vi "solar_voy TCP Listener Wait.vi"(7 "Instance":i32, 8 "error in (no error)":errorcluster, 9 "timeout ms (-1)":i32=-1, 10 "Listener ID":refnum<k5>, 11 "Voyager Refnum in":T1) -> (0 "error out":errorcluster, 2 "Connection ID":refnum<k5>, 3 "Voyager Refnum out":T1)   [LabVIEW 2018]
doc: "This waits for a single TCP client connection."
uses:
  solar_voy_ctl Voyager Refnum.ctl
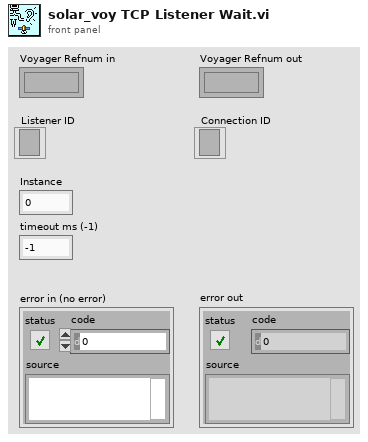
[diagram p1: front panel]
types:
  T1 = typedef "solar_voy_ctl Voyager Refnum.ctl" = refnum<k1>
  T2 = typedef "solar_voy_ctl Voyager.ctl" = cluster{"PACKETS":T3[], "COSMOS_Root":path, "CMD_HDR":T8, "TLM_HDR":T8, "TCPs":T9[], "VoyagerIDOffset":cluster{"VoyagerIDOffset":u16[], "Target Names":string[]}}
  T3 = typedef "solar_voy_def_ctl PACKET.ctl" = cluster{"PACKET_ID":T4, "ENDIAN":enum8{"BIG", "LITTLE"}, "DESC":string, "HZRD":bool, "ITEMS":T5[], "NoExport":bool, "last_time":timestamp, "last_count":u32, "last_data":string}
  T4 = typedef "solar_voy_def_ctl PACKET_ID.ctl" = cluster{"ID":u16, "CMD":enum8{"CMD", "TLM"}, "TARGET":string, "PACKET":string}
  T5 = typedef "solar_voy_def_ctl ITEM.ctl" = cluster{"NAME":string, "OFFSET":i32, "SIZE":i32, "TYPE":T6, "EACH_SIZE":i32, "LVTYPE":T7, "MIN":dbl, "MAX":dbl, "DEFAULT":string, "DESC":string, "ID":bool, "MODIFIERS":variant, "last_value":variant}
  T6 = typedef "solar_voy_def_ctl ITEM TYPE.ctl" = enum8{"BLOCK", "INT", "UINT", "FLOAT", "STRING"}
  T7 = typedef "solar_type Item Type.ctl" = enum16{"NULL", "UNKNOWN", "CLUSTER", "I8", "I16", "I32", "I64", "U8", "U16", "U32", "U64", "U8_ENUM", "U16_ENUM", "U32_ENUM", "SGL", "DBL", "BOOLEAN", "STRING", "PATH", "VISA", "TAG", "TIME", "I8_1D", "I16_1D", "I32_1D", "I64_1D", "U8_1D", "U16_1D", "U32_1D", "U64_1D", "U8_ENUM_1D", "U16_ENUM_1D", "U32_ENUM_1D", "SGL_1D", "DBL_1D", "BOOLEAN_1D", "STRING_1D", "PATH_1D", "VISA_1D", "TAG_1D", "TIME_1D", "I8_2D", "I16_2D", "I32_2D", "I64_2D", "U8_2D", "U16_2D", "U32_2D", "U64_2D", "U8_ENUM_2D", "U16_ENUM_2D", "U32_ENUM_2D", "SGL_2D", "DBL_2D", "BOOLEAN_2D", "STRING_2D", "PATH_2D", "VISA_2D", "TAG_2D", "TIME_2D"}
  T8 = typedef "solar_voy_def_ctl HDR.ctl" = cluster{"ITEMS":T5[], "LENGTH_NAME":string, "LENGTH_VALUE_OFFSET":i32, "ID_NAME":string, "ENDIAN":enum8{"BIG", "LITTLE"}, "GUID_NAME":string, "DEFAULT_TARGET":string, "DEFAULT_PACKET":string, "DEFAULT_ERROR":string}
  T9 = typedef "solar_voy_ctl TCP.ctl" = cluster{"Connected":bool, "Port":u16, "Listener":refnum<k5>, "ServerIP":string, "TCP":refnum<k5>, "Setup":T10, "VIRefnum":refnum<vi>, "TARGETS_CMD":string[], "TARGETS_TLM":string[]}
  T10 = typedef "solar_voy_ctl Port Setup.ctl" = enum8{"SERVER", "CLIENT", "SERVER_CMD", "SERVER_TLM"}
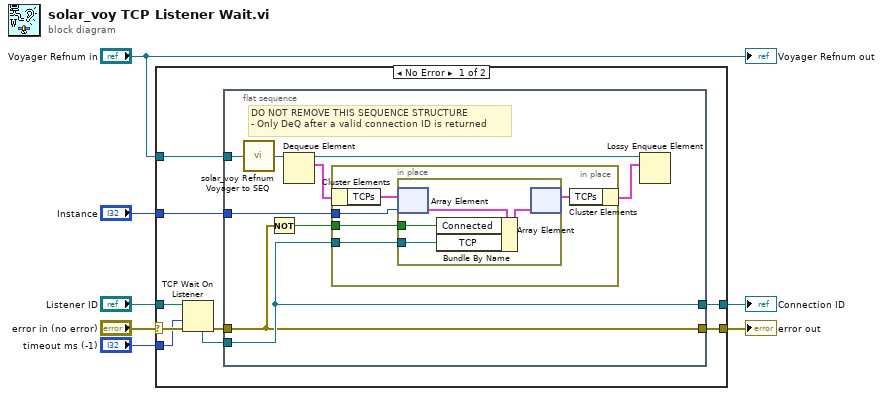
[diagram p0: block diagram]
diagram:
  n1 = case shown="No Error" "error in (no error)" {
    selector: "error in (no error)" -> [w11 w35]
    tunnel: [w16 _] -> w7
    tunnel: "Instance" -> [w14 _]
    tunnel: "Listener ID" -> [w12 _]
    tunnel: [w10 w35] -> w3
    tunnel: "Voyager Refnum in" -> [w9 _]
    tunnel: "timeout ms (-1)" -> [w8 _]
    frame No Error {
      n2 = TCP Wait On Listener(8:w11, 9:w8, 11:w12) -> (0:w15:errorcluster, 4:w13:refnum<k5>)  [unwired: 4 out]
      n3 = flat-sequence {
        tunnel: w13 -> [w21]
        tunnel: w14 -> [w25]
        tunnel: w9 -> [w22]
        tunnel: w15 -> [w20]
        tunnel: [w20] -> w10
        tunnel: [w21] -> w16
        frame #0 {
          # "DO NOT REMOVE THIS SEQUENCE STRUCTURE\n- Only DeQ after a valid connection ID is returned"
          n4 = call "solar_voy Refnum Voyager to SEQ.vi"("Voyager Refnum"=w22) -> ("Voyager SEQ"=w24:refnum<queue>)
          n5 = Not(x=w20) -> (.not. x?=w19:bool)
          n6 = Dequeue Element(queue=w24) -> (queue out=w23:refnum<queue>, element=w18:T2)  [unwired: 2 in, 2 out]
          n7 = in-place {
            in-place-border: w25 -> [w30]
            in-place-border: w21 -> [w29]
            in-place-border: w19 -> [w28]
            n8 = in-place-cluster #1(w18) -> ("TCPs"=w27:T9[])
            n9 = in-place {
              in-place-border: w29 -> [w32]
              in-place-border: w28 -> [w31]
              n10 = in-place-array #2(w27, w30) -> (w34:T9)
              n11 = Bundle By Name(cluster=w34, "Connected"=w31, "TCP"=w32) -> (w33:T9)
              n12 = in-place-array #2(w33) -> (w26:T9[])  [unwired: 1 out]
            }
            n13 = in-place-cluster #1("TCPs"=w26) -> (w17:T2)
          }
          n14 = Lossy Enqueue Element(queue=w23, element=w17) -> ()  [unwired: 1 in, 4 out]
        }
      }
    }
    frame Error {
    }
  }
  "Connection ID" <- w7
  "error out" <- w3
  "Voyager Refnum out" <- "Voyager Refnum in"
